vi "EXA shm ack Command exit Control LV.vi"(8 "error in (no error)":errorcluster, 11 "ackcmd_Ctl":T1) -> (0 "error out":errorcluster, 2 "function return":i32, 3 "ackcmd_Ctl out":T1)   [LabVIEW 2016, in "SALLV_EXA.lvlib"]
doc: "int EXA_shm_ackCommand_exitControlLV(EXA_ackcmdLV *ackcmd_Ctl);"
uses:
  SALLV_EXA.lvlib
  SALLV_EXA.so
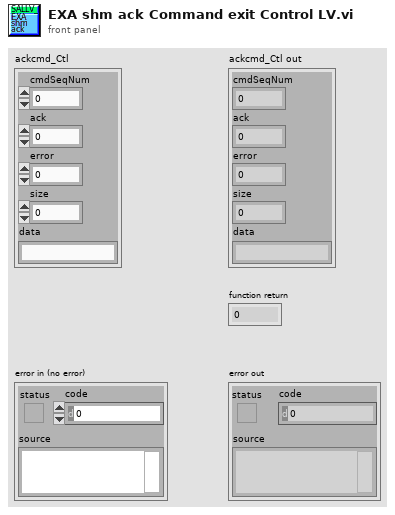
[diagram p1: front panel]
types:
  T1 = cluster{"cmdSeqNum":i32, "ack":i32, "error":i32, "size":i32, "data":string}
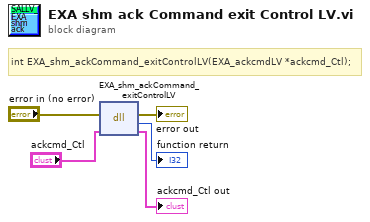
[diagram p0: block diagram]
diagram:
  # "int EXA_shm_ackCommand_exitControlLV(EXA_ackcmdLV *ackcmd_Ctl);"
  n1 = dll-call lib="home/plotz/SALLV_EXA/SALLV_EXA.*" fn="EXA_shm_ackCommand_exitControlLV"(error in="error in (no error)", "ackcmd_Ctl"="ackcmd_Ctl") -> (error out=→"error out":errorcluster, →"function return":i32, "ackcmd_Ctl"=→"ackcmd_Ctl out":T1)  [unwired: 2 in, 1 out]
